vi "ISX3_Cmd_GetSyncTime.vi"() -> (0 "Get SyncTimeCmd":u8[](array[numeric]))   [LabVIEW 2012, in "Sciospec ISX3 Impedance Analyzer.lvlib"]
uses:
  Sciospec ISX3 Impedance Analyzer.lvlib
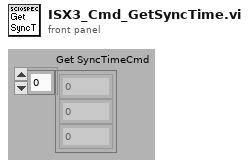
[diagram p1: front panel]
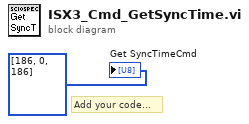
[diagram p0: block diagram]
diagram:
  # "Add your code..."
  "Get SyncTimeCmd" <- u8[] [186, 0, 186]
